vi "Example - Event-based operations.vi"() -> ()   [LabVIEW 2020, in "wamplv.lvlib"]
uses:
  wamplv.lvlib
  WAMP Client/WAMP Client.lvclass
  de229235-2a3a-4925-9c3f-b8af0efd4371.vi
  699b3d9d-c32a-421f-a194-d91978fc0265.vi
  aa2eb0e7-7d03-3fef-44a9-bd5fee1bda3f.vi
  WAMP Client/API/WAMP/JSON/Call JSON.vi
  WAMP Client/API/WAMP/JSON/Publish JSON.vi
panel:
  in  "RPC return value":string="hello back"
  in  "RPC Name":string="test.topic"
  in  "Register RPC":bool caption="Publish Topic"
  out "Error URI":string
  out "Callee Error?":bool
  out "Call Result ArgumentKw":string
  out "Call Result Arguments":string
  in  "Call Arguments":string[](array[string])=["Hello!"]
  in  "Call URI":string="test.topic"
  in  "Call":bool caption="Publish Topic"
  in  "Unsubscribe":bool caption="Publish Topic"
  out "Topic:":string
  out "ArgumentKw Payload":string
  out "Arguments Payload":string
  out "Event received on:":string
  in  "Publish Argument Payload":string[](array[string])
  in  "Subscription URI":string="test.topic"
  in  "Subscribe":bool caption="Publish Topic"
  in  "Disconnect":bool caption="Publish Topic"
  in  "Realm":string="default_realm"
  in  "Topic URI":string="test.topic"
  in  "Publish":bool caption="Publish Topic"
  in  "Router Address":string="ws://localhost:8080/"
  # "The router URI must a fully-formed URI: \n\ntcp://localhost:8080/ (RawSocket TCP)\ntcps://localhost:8080/ (RawSocket TCP with TLS/SSL)\nws://localhost:8080/ (WebScoket)\nws://localhost:8080/ws (WebScoket)\nwss://localhost:8080/ (WebSocket TCP with TLS/SSL)\n\nAlways disconnect by pressing the disconnect button, not by aborting the VI. Otherwise the \nWAMP session will conitinue in the background."
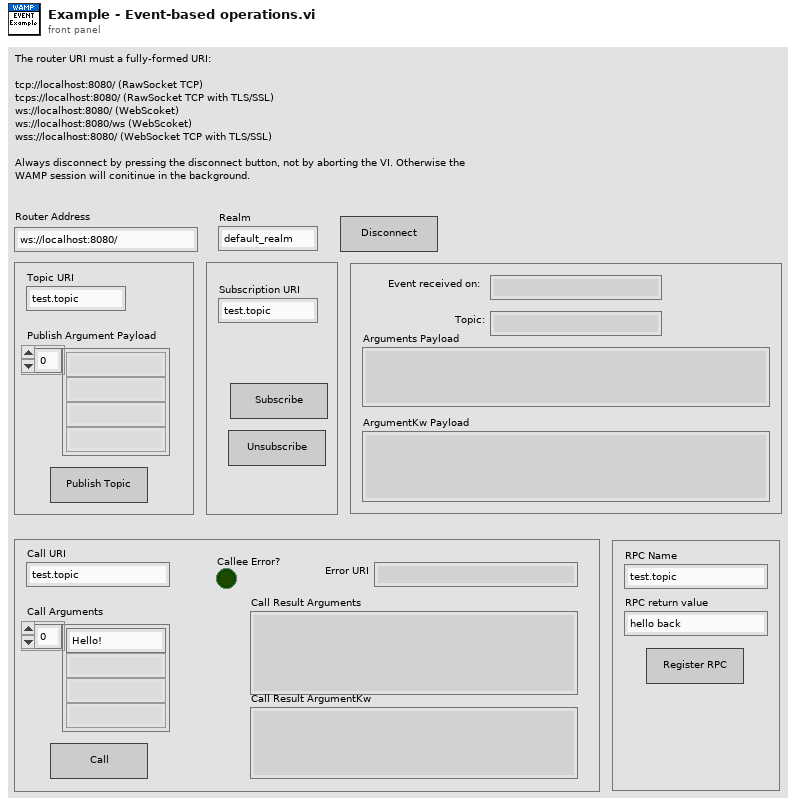
[diagram p1: front panel]
types:
  T1 = typedef "wamplv.lvlib/Error or abort detail (JSON).ctl" = cluster{"URI":string, "Arguments Payload":string, "ArgumentKw Payload":string, "Details":string, "Associated LabVIEW Error":errorcluster}
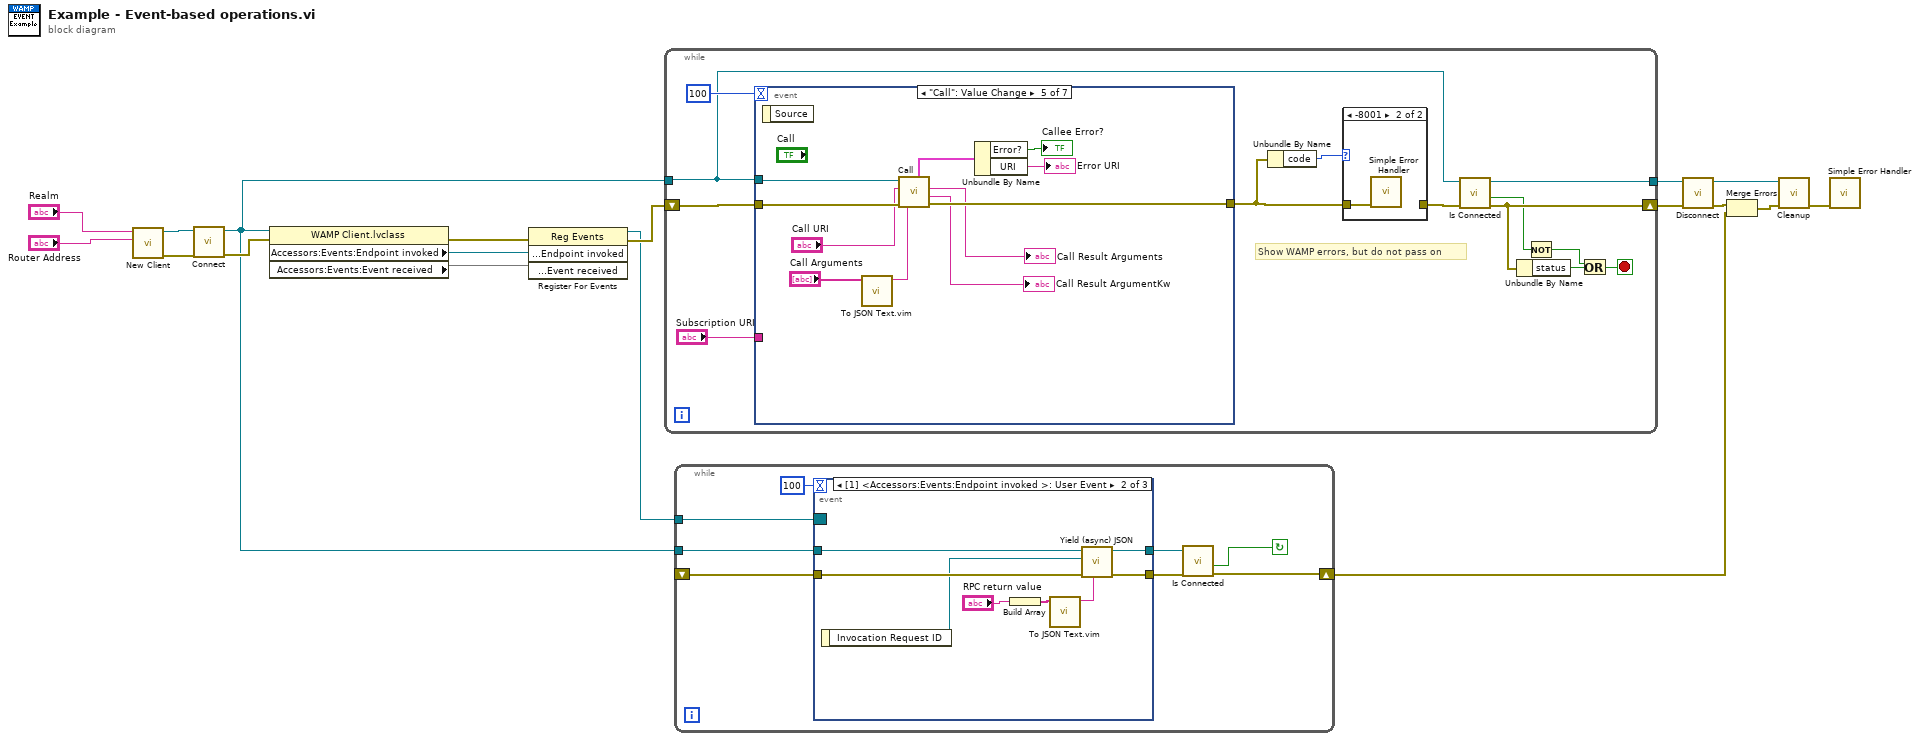
[diagram p0: block diagram]
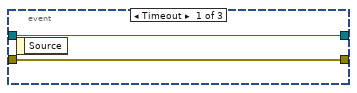
[diagram p2: hidden frame]
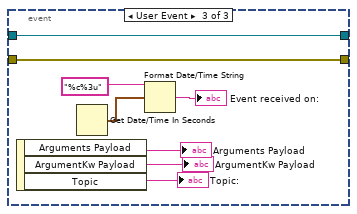
[diagram p3: hidden frame]
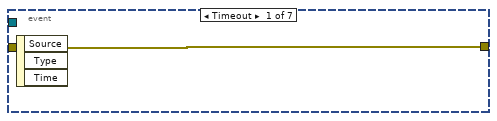
[diagram p5: hidden frame]
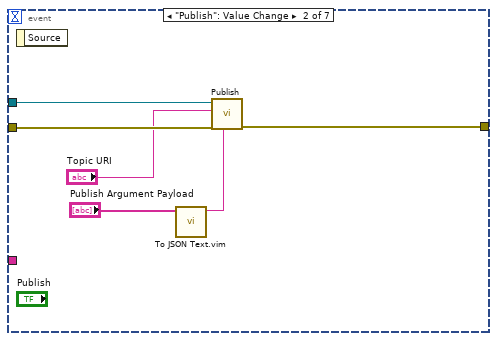
[diagram p6: hidden frame]
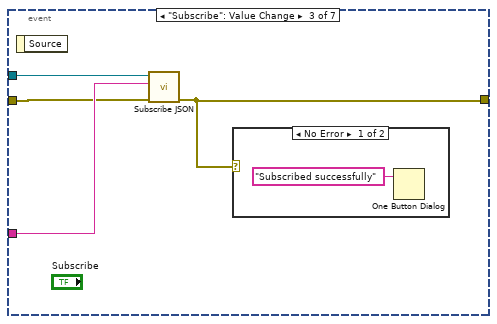
[diagram p7: hidden frame]
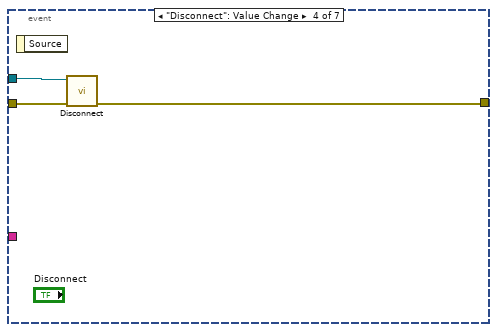
[diagram p9: hidden frame]
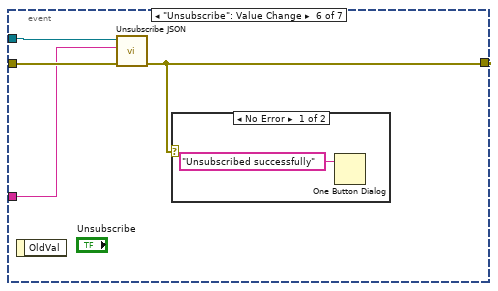
[diagram p10: hidden frame]
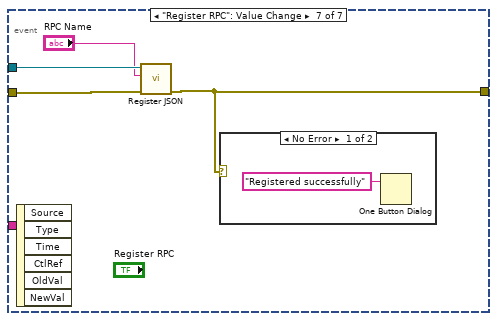
[diagram p12: hidden frame]
diagram:
  n1 = call "New Client.vi"("Address"="Router Address", "Realm"="Realm") -> ("error out"=w15:errorcluster, "WAMP client out"=w16:refnum<class "WAMP Client.lvclass">)  [unwired: 8 in]
  n2 = call "Connect.vi"("error in"=w15, "WAMP Client in"=w16) -> ("error out"=w12:errorcluster, "WAMP Client out"=w9:refnum<class "WAMP Client.lvclass">)  [unwired: 8 in]
  n3 = property class="WAMP Client.lvclass"(reference=w9, error in=w12) -> (error out=w7:errorcluster, "Accessors:Events:Endpoint invoked "=w6:refnum<user-event>, "Accessors:Events:Event received "=w5)  [unwired: 1 out]
  n4 = register-events(error in=w7, w6, w5) -> (reference out=w10:refnum<event-registration>, error out=w11:errorcluster)  [unwired: 1 in]
  n5 = while {
    tunnel: w9 -> [w25]
    shift-right: [w23] -> w14
    shift-left: w11 -> [w31]
    tunnel: [w24] -> w13
    stop <- w21 stop-if-true
    # "Show WAMP errors, but do not pass on"
    n6 = event shown="[4] \"Call\": Value Change" {
      selector: _ -> [_ _ _ _ _ _ _]
      dyn-events: _ -> [_ _ _ _ _ _ _]
      timeout: 100 -> [_ _ _ _ _ _ _]
      tunnel: w25 -> [_ w38 w44 w48 w59 w62 w68]
      tunnel: w31 -> [w34 w39 w42 w47 w58 w63 w67]
      tunnel: [w34 w36 w41 w46 w56 w60 w66] -> w27
      tunnel: "Subscription URI" -> [_ _ w43 _ _ w61 _]
      event Timeout {
        n7 = event-data() -> ()  [unwired: 1 in, 3 out]
      }
      event "Publish": Value Change {
        n8 = event-data() -> ()  [unwired: 1 in, 1 out]
        n9 = call "To JSON Text.vim"("Anything"="Publish Argument Payload") -> ("<JSON>"=w37:string)  [unwired: 9 in, 1 out]
        n10 = call-poly "Publish.vi"("Arguments"=w37, "Error in"=w39, "Topic"="Topic URI", "WAMP Client in"=w38) -> ("Error out"=w36:errorcluster)  [unwired: 5 in, 2 out]
      }
      event "Subscribe": Value Change {
        n11 = event-data() -> ()  [unwired: 1 in, 1 out]
        n12 = call-dynamic "Subscribe JSON.vi"("error in (no error)"=w42, "Topic"=w43, "WAMP Client in"=w44) -> ("error out"=w41:errorcluster)  [unwired: 4 in, 4 out]
        n13 = case shown="No Error" w41 {
          frame No Error {
            n14 = One Button Dialog(message="Subscribed successfully") -> ()  [unwired: 1 in, 1 out]
          }
          frame Error {
          }
        }
      }
      event "Disconnect": Value Change {
        n15 = event-data() -> ()  [unwired: 1 in, 1 out]
        n16 = call-dynamic "Disconnect.vi"("error in"=w47, "WAMP Client in"=w48) -> ("error out"=w46:errorcluster)  [unwired: 8 in, 1 out]
      }
      event "Call": Value Change {
        n17 = event-data() -> ()  [unwired: 1 in, 1 out]
        n18 = call "To JSON Text.vim"("Anything"="Call Arguments") -> ("<JSON>"=w53:string)  [unwired: 9 in, 1 out]
        n19 = call-poly "Call.vi"("Arguments"=w53, "Error in"=w58, "Topic URI"="Call URI", "WAMP Client in"=w59) -> ("Error out"=w56:errorcluster, "ArgumentKw Payload"=→"Call Result ArgumentKw":string, "Arguments Payload"=→"Call Result Arguments":string, "WAMP Error"=w51:T1)  [unwired: 3 in, 1 out]
        n20 = Unbundle By Name(w51) -> ("Error?"=→"Callee Error?":bool, "URI"=→"Error URI":string)
      }
      event "Unsubscribe": Value Change {
        n21 = event-data() -> ()  [unwired: 1 in, 1 out]
        n22 = call-dynamic "Unsubscribe JSON.vi"("error in (no error)"=w63, "Topic"=w61, "WAMP Client in"=w62) -> ("error out"=w60:errorcluster)  [unwired: 7 in, 1 out]
        n23 = case shown="No Error" w60 {
          frame No Error {
            n24 = One Button Dialog(message="Unsubscribed successfully") -> ()  [unwired: 1 in, 1 out]
          }
          frame Error {
          }
        }
      }
      event "Register RPC": Value Change {
        n25 = event-data() -> ()  [unwired: 1 in, 6 out]
        n26 = call-dynamic "Register JSON.vi"("Error in"=w67, "Procedure URI"="RPC Name", "WAMP Client in"=w68) -> ("Error out"=w66:errorcluster)  [unwired: 6 in, 2 out]
        n27 = case shown="No Error" w66 {
          frame No Error {
            n28 = One Button Dialog(message="Registered successfully") -> ()  [unwired: 1 in, 1 out]
          }
          frame Error {
          }
        }
      }
    }
    n29 = Unbundle By Name(w27) -> ("code"=w28:i32)
    n30 = case shown="-8001" w28 {
      tunnel: w27 -> [w32 w33]
      tunnel: [w32 _] -> w26
      frame 0, Default {
      }
      frame -8001 {
        n31 = call <vilib>:"Simple Error Handler.vi"("error in (no error)"=w33) -> ()  [unwired: 4 in, 5 out]
      }
    }
    n32 = call "Is Connected.vi"("error in"=w26, "WAMP Client in"=w25) -> ("error out"=w23:errorcluster, "Is Connected?"=w22:bool, "WAMP Client out"=w24:refnum<class "WAMP Client.lvclass">)  [unwired: 7 in]
    n33 = Unbundle By Name(w23) -> ("status"=w19:bool)
    n34 = Not(x=w22) -> (.not. x?=w20:bool)
    n35 = Or(x=w20, y=w19) -> (x .or. y?=w21:bool)
  }
  n36 = while {
    tunnel: w10 -> [w77]
    tunnel: w9 -> [w76]
    shift-right: [w72] -> w8
    shift-left: _ -> [w71]
    stop <- w73 continue-if-true
    n37 = event shown="[1] <Accessors:Events:Endpoint invoked >: User Event" {
      selector: w77 -> [_ _ _]
      dyn-events: _ -> [_ _ _]
      timeout: 100 -> [_ _ _]
      tunnel: w76 -> [w79 w84 w89]
      tunnel: [w78 w83 w88] -> w75
      tunnel: [w79 w82 w89] -> w74
      tunnel: w71 -> [w78 w81 w88]
      event Timeout {
        n38 = event-data() -> ()  [unwired: 1 in, 1 out]
      }
      event User Event {
        n39 = event-data() -> ("Invocation Request ID"=w80:refnum<class "Invocation Request ID.lvclass">)  [unwired: 1 in]
        n40 = Build Array("RPC return value") -> (w85:string[])
        n41 = call "To JSON Text.vim"("Anything"=w85) -> ("<JSON>"=w86:string)  [unwired: 9 in, 1 out]
        n42 = call "Yield (async) JSON.vi"("Arguments"=w86, "error in (no error)"=w81, "Invocation Request"=w80, "WAMP Client in"=w84) -> ("error out"=w83:errorcluster, "WAMP Client out"=w82:refnum<class "WAMP Client.lvclass">)  [unwired: 6 in]
      }
      event User Event {
        n43 = event-data() -> ("Arguments Payload"=→"Arguments Payload":string, "ArgumentKw Payload"=→"ArgumentKw Payload":string, "Topic"=→"Topic:":string)  [unwired: 1 in]
        n44 = Get Date/Time In Seconds() -> (seconds since 1Jan1904=w94:timestamp)
        n45 = Format Date/Time String(time format string (%c)="%c%3u", seconds (now)=w94) -> (date/time string=→"Event received on:":string)  [unwired: 1 in]
      }
    }
    n46 = call "Is Connected.vi"("error in"=w75, "WAMP Client in"=w74) -> ("error out"=w72:errorcluster, "Is Connected?"=w73:bool)  [unwired: 7 in, 1 out]
  }
  n47 = call-dynamic "Disconnect.vi"("error in"=w14, "WAMP Client in"=w13) -> ("error out"=w2:errorcluster, "WAMP Client out"=w4:refnum<class "WAMP Client.lvclass">)  [unwired: 8 in]
  n48 = Merge Errors(w2, w8) -> (w1:errorcluster)
  n49 = call-dynamic "Cleanup.vi"("error in"=w1, "WAMP Client in"=w4) -> ("error out"=w3:errorcluster)  [unwired: 8 in, 1 out]
  n50 = call <vilib>:"Simple Error Handler.vi"("error in (no error)"=w3) -> ()  [unwired: 4 in, 5 out]
